vi "SoC1.vi"(3 "Coefficients":dbl[](array[numeric]), 4 "Time":i32, 5 "BAT Current (A)":dbl) -> (0 "Time (min)":i32, 1 "State":string, 2 "SoC (%)":i32)   [LabVIEW 2015]
uses:
  <vilib>/Analysis/polynomials.llb/Polynomial Roots (DBL).vi
  <vilib>/Analysis/NI_AALPro.lvlib
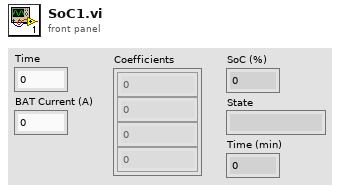
[diagram p1: front panel]
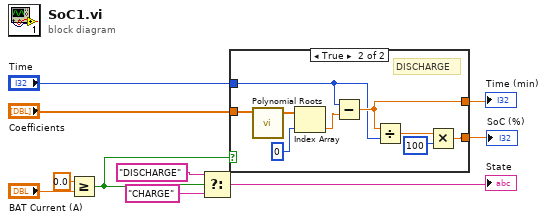
[diagram p0: block diagram]
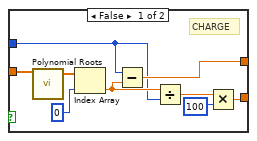
[diagram p2: hidden frame]
diagram:
  n1 = Greater Or Equal?(x=0.0, y="BAT Current (A)") -> (x >= y?=w7:bool)
  n2 = Select(t="DISCHARGE" ("f"), s=w7, f="CHARGE" ("t")) -> (s? t:f=→"State":string)
  n3 = case shown="True" w7 {
    tunnel: [w15 w23] -> w4
    tunnel: [w14 w22] -> w5
    tunnel: "Coefficients" -> [w12 w21]
    tunnel: "Time" -> [w11 w20]
    frame False {
      # "CHARGE"
      n4 = call-poly <vilib>:"Polynomial Roots.vi"("P(x)"=w12) -> ("Roots"=w19:cdb[])  [unwired: 9 in, 1 out]
      n5 = Index Array(array=w19, index=0) -> (element=w13:cdb)
      n6 = Subtract(x=w11, y=w13) -> (x-y=w15:cdb)
      n7 = Divide(x=w13, y=w11) -> (x/y=w18:cdb)
      n8 = Multiply(x=w18, y=100) -> (x*y=w14:cdb)
    }
    frame True {
      # "DISCHARGE"
      n9 = call-poly <vilib>:"Polynomial Roots.vi"("P(x)"=w21) -> ("Roots"=w24:cdb[])  [unwired: 9 in, 1 out]
      n10 = Index Array(array=w24, index=0) -> (element=w28:cdb)
      n11 = Subtract(x=w20, y=w28) -> (x-y=w23:cdb)
      n12 = Divide(x=w23, y=w20) -> (x/y=w27:cdb)
      n13 = Multiply(x=w27, y=100) -> (x*y=w22:cdb)
    }
  }
  "Time (min)" <- w4
  "SoC (%)" <- w5
